vi "Combine Data Array.vi"(8 "Num. elements":i32, 9 "Index data":dbl[](array[numeric]), 10 "Pressure data":dbl[][](array[numeric])) -> (2 "All data":dbl[][](array[numeric]))   [LabVIEW 2013]
doc: "This sub-VI combines pressure data (5 rows by 2000 columns) and index data (run time, command, pressure reading, temperature readings) into a single big data set by duplicating index values for each unique pressure reading at this loop iteration, combining data sets, and transposing. The result is a data set with columns [time, air command, pilot command, inner command, outer command, pressure reading, T1, T2, T3, T4, dynP1, dynP2, dynP3, dynP4, dynP5] 2000 rows long."
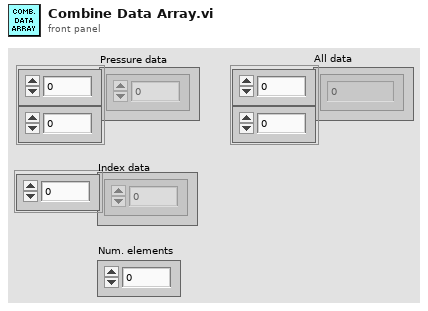
[diagram p1: front panel]
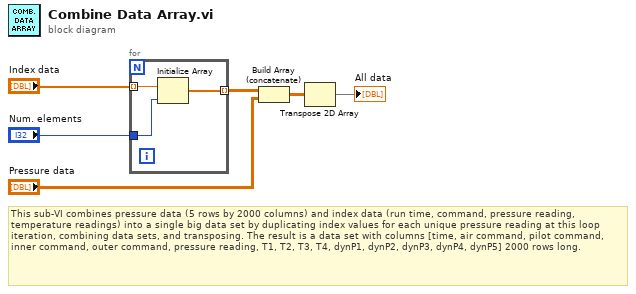
[diagram p0: block diagram]
diagram:
  # "This sub-VI combines pressure data (5 rows by 2000 columns) and index data (run time, command, pressure reading, temperature readings) into a single big data set by duplicating index values for each unique pressure reading at this loop iteration, combining data sets, and transposing. The result is a data set with columns [time, air command, pilot command, inner command, outer command, pressure reading, T1, T2, T3, T4, dynP1, dynP2, dynP3, dynP4, dynP5] 2000 rows long."
  n1 = for {
    tunnel: "Index data" -> [w9] mode=indexing
    tunnel: "Num. elements" -> [w8]
    tunnel: [w7] -> w3 mode=indexing
    n2 = Initialize Array(w9, w8) -> (w7:dbl[])
  }
  n3 = Build Array (concatenate)(w3, "Pressure data") -> (w1:dbl[][])
  n4 = Transpose 2D Array(2D array=w1) -> (transposed array=→"All data":dbl[][])
